vi "Setup subWorker - Second Level Worker.vi"(8 "error in":errorcluster, 11 "First Level Worker in":refnum<class "First Level Worker.lvclass">) -> (0 "error out":errorcluster, 3 "First Level Worker out":refnum<class "First Level Worker.lvclass">)   [LabVIEW 2017, in "Method 1.lvlib" / "First Level Worker.lvclass"]
doc: "This VI sets up the framework parameters of a statically-linked subWorker."
uses:
  First Level Worker.lvclass
  First Level Worker.lvclass/First Level Worker.ctl
  Second Level Worker/Second Level Worker.lvclass
  C:/Program Files (x86)/National Instruments/LabVIEW 2017/vi.lib/addons/_Workers/Library/Classes/Worker/Worker.lvclass
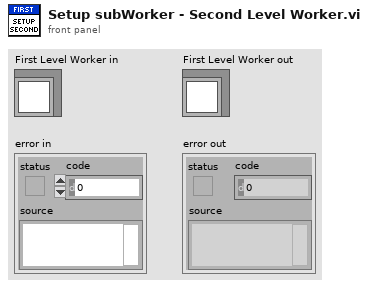
[diagram p1: front panel]
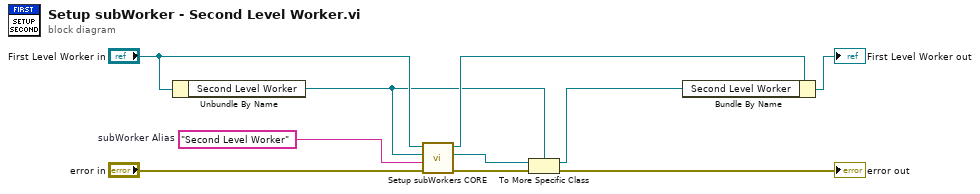
[diagram p0: block diagram]
diagram:
  w6 = "Second Level Worker"  # subWorker Alias
  n1 = Unbundle By Name("First Level Worker in") -> ("Second Level Worker"=w3:refnum<class "Second Level Worker.lvclass">)
  n2 = call-dynamic "Setup subWorkers CORE.vi"("error in"="error in", "subWorker Alias"=w6, "subWorker"=w3, "Worker"="First Level Worker in") -> ("error out"=w5:errorcluster, "subWorker out"=w1:refnum<class "Worker.lvclass">, "Worker out"=w8:refnum<class "First Level Worker.lvclass">)  [unwired: 5 in]
  n3 = To More Specific Class(target class=w3, reference=w1, error in=w5) -> (specific class reference=w2:refnum<class "Second Level Worker.lvclass">, error out=→"error out":errorcluster)
  n4 = Bundle By Name(cluster=w8, "Second Level Worker"=w2) -> (→"First Level Worker out":refnum<class "First Level Worker.lvclass">)
